vi "main.vi"(8 "Error in":errorcluster) -> (0 "error out":errorcluster)   [LabVIEW 2018, in "Controller.lvlib"]
doc: "The main VI of the module."
uses:
  Controller.lvlib
  vi/Module Queue Actions.ctl
  ctl/Module State--enum.ctl
  Common/Common.lvlib
  Common/ctl/Stop all modules states--enum.ctl
  Error Handler/Error Handler.lvlib
  Error Handler/ctl/Module State--enum.ctl
  Error Handler/ctl/Error source--enum.ctl
  Common/ctl/Error to pass.ctl
  Display Console/Simulated/Display Console.lvlib
  Sensor Interface/Simulated/Sensor Interface.lvlib
  User Console/Simulated/User Console.lvlib
  User Console/Simulated/ctl/Module State--enum.ctl
  vi/Module Data.ctl
  ctl/Module Data--cluster.ctl
  User Console/Simulated/ctl/control enable states--cluster.ctl
  Sensor Interface/Simulated/ctl/Module State--enum.ctl
  Display Console/Simulated/ctl/Module State--enum.ctl
  vi/state--global.vi
  ctl/Config db action--enum.ctl
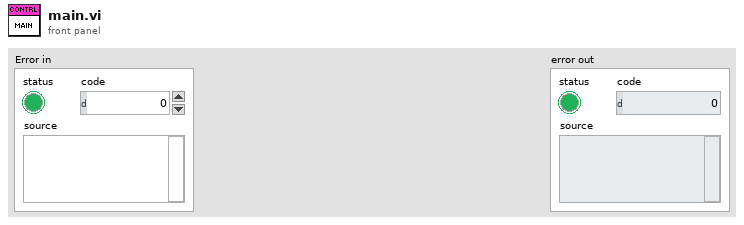
[diagram p1: front panel]
types:
  T1 = typedef "Controller.lvlib/Module Data--cluster.ctl" = cluster{"Atm messages":T2[], "No. incorrect login attempts":i32, "Balance":dbl}
  T2 = typedef "Controller.lvlib/Module Data.ctl" = cluster{"message name":string, "message text":string}
  T3 = typedef "Controller.lvlib/Module Queue Actions.ctl" = enum16{"Create", "Get", "Destroy"}
  T4 = typedef "Common.lvlib/Stop all modules states--enum.ctl" = enum16{"Create", "Get", "Send 'Stop all' Message", "Destroy"}
  T5 = typedef "Controller.lvlib/Module State--enum.ctl" = enum16{"Init", "Error", "Close", "User Console: Card Reader Pressed", "Sensor Interface: Deposit Received pressed", "Sensor Interface: Funds Dispensed Pressed", "Idle", "Login State", "Balance Enquiry", "Deposit State", "Withdrawal State", "Fast Cash State", "Configuration Database", "Inactivity Timeout", "Terminate State", "Wait for account number", "Verify account number", "Wait for new transaction button"}
  T6 = typedef "Common.lvlib/Error source--enum.ctl" = enum16{"Display Console", "User Console", "Sensor Interface IO", "Process Step", "Other"}
  T7 = typedef "Common.lvlib/Error to pass.ctl" = cluster{"Error source":T6, "Error":errorcluster}
  T8 = typedef "Error Handler.lvlib/Module State--enum.ctl" = enum16{"Init", "Error", "Idle", "Close", "Handle External Error", "Log to file"}
  T9 = typedef "User Console.lvlib/Module State--enum.ctl" = enum16{"Init", "Error", "Idle", "Close", "Transaction Button Pressed: Which?", "Balance Inquiry Pressed", "Desposit Pressed", "Withdrawal Pressed", "Fast Cash Pressed", "New Transaction Pressed", "Terminate Session Pressed", "Card Reader Pressed", "Keypad Button Pressed", "Update Keypad Screen", "Enable/disable controls", "Card reader: On?"}
  T10 = typedef "Display Console.lvlib/Module State--enum.ctl" = enum16{"Init", "Error", "Idle", "Close", "Card Read LED", "Update Message Screen", "Update Current Transaction", "Enable/disable controls"}
  T11 = typedef "Sensor Interface.lvlib/Module State--enum.ctl" = enum16{"Init", "Error", "Idle", "Close", "Enable/disable controls"}
  T12 = typedef "Controller.lvlib/Config db action--enum.ctl" = enum16{"Read", "Search", "Write"}
  T13 = typedef "User Console.lvlib/control enable states--cluster.ctl" = cluster{"Transactions":enum8{"Enabled", "Disabled", "Disabled and Grayed Out"}, "Card reader":enum8{"Enabled", "Disabled", "Disabled and Grayed Out"}, "Keypad":enum8{"Enabled", "Disabled", "Disabled and Grayed Out"}}
  T14 = typedef "Module Data.ctl" = cluster{"message name":string, "message text":string}
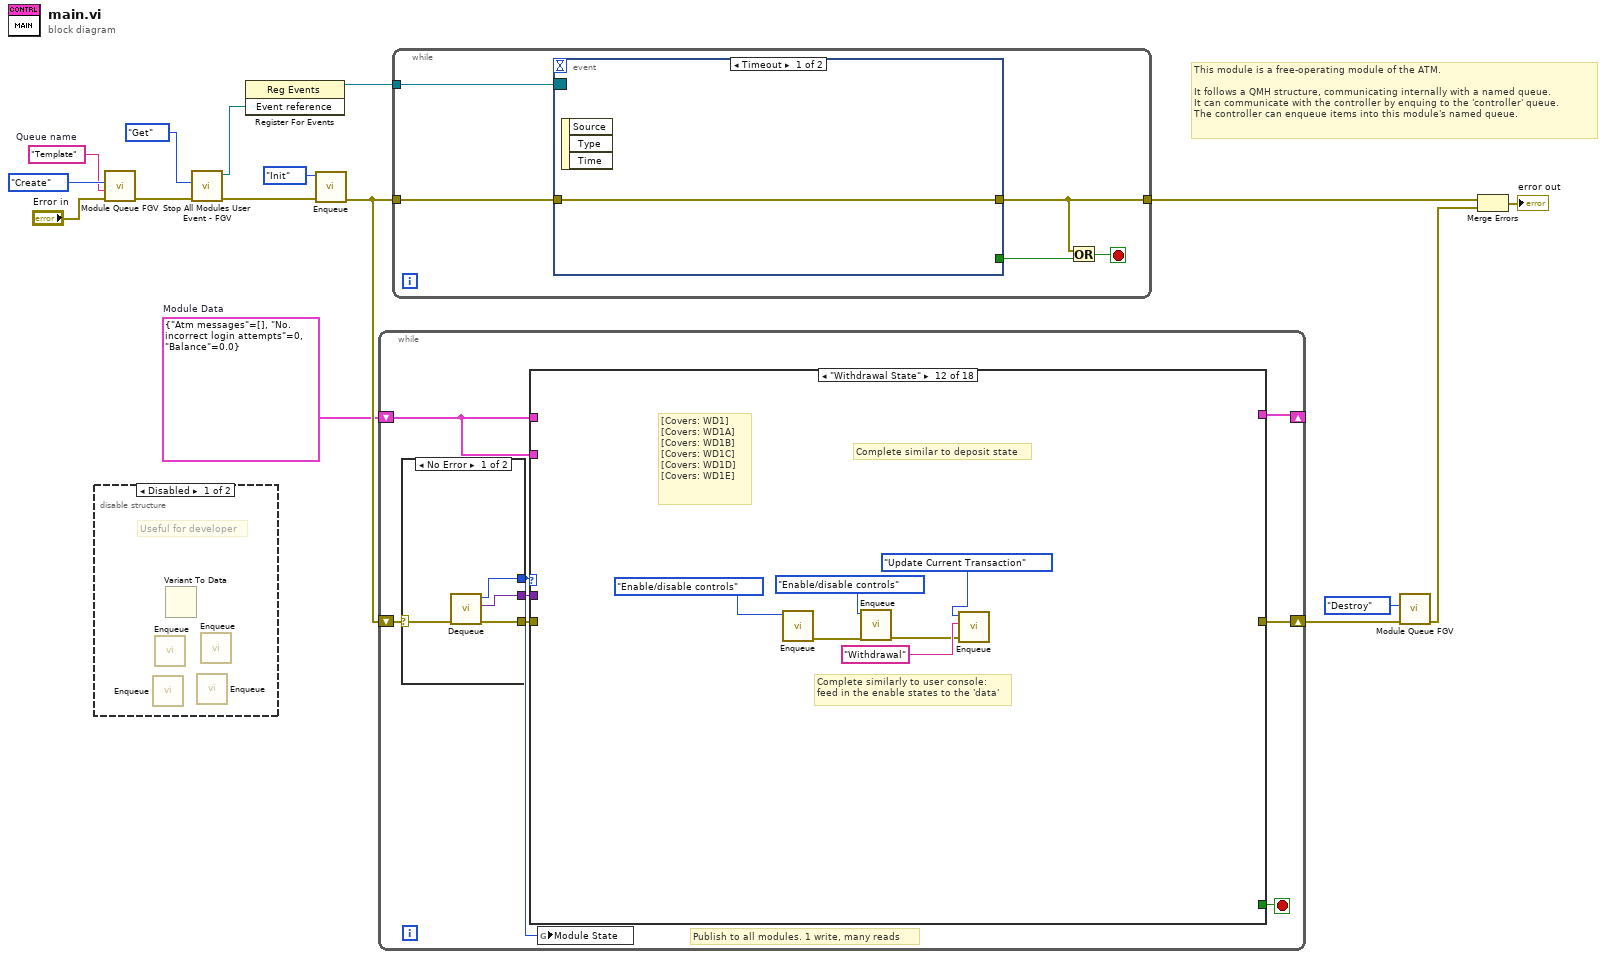
[diagram p0: block diagram]
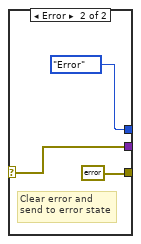
[diagram p3: hidden frame]
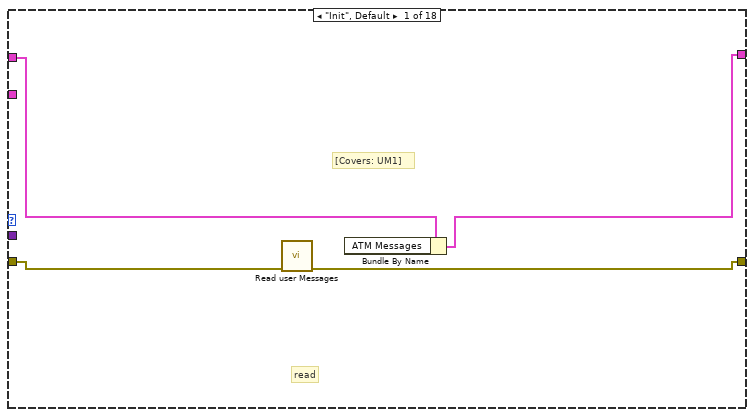
[diagram p4: hidden frame]
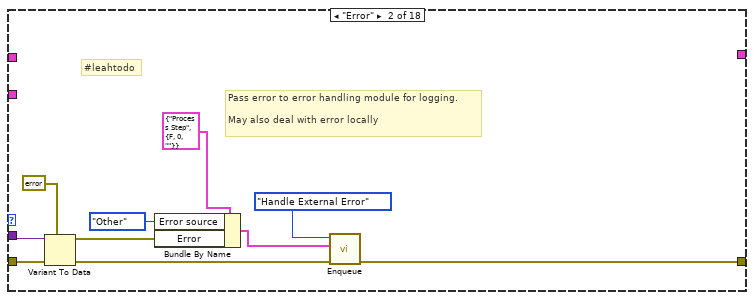
[diagram p5: hidden frame]
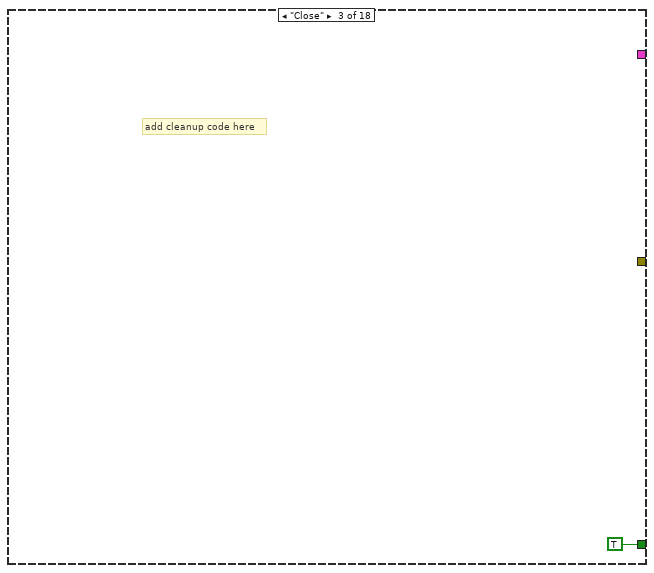
[diagram p6: hidden frame]
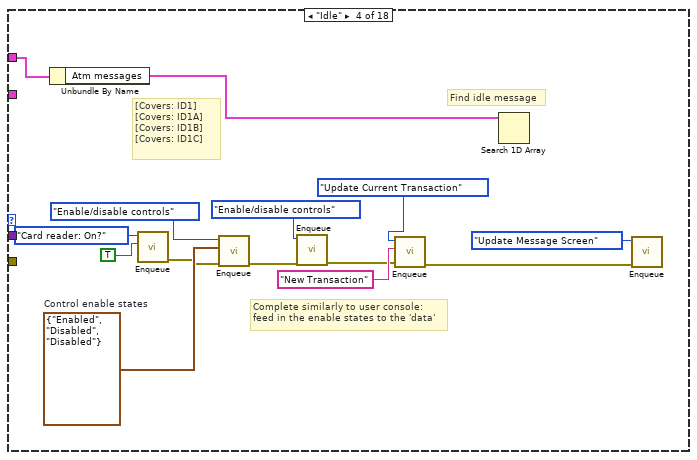
[diagram p7: hidden frame]
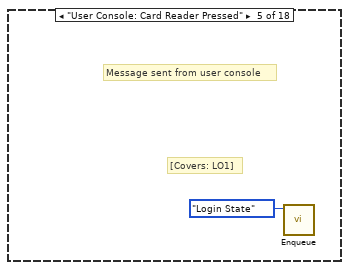
[diagram p8: hidden frame]
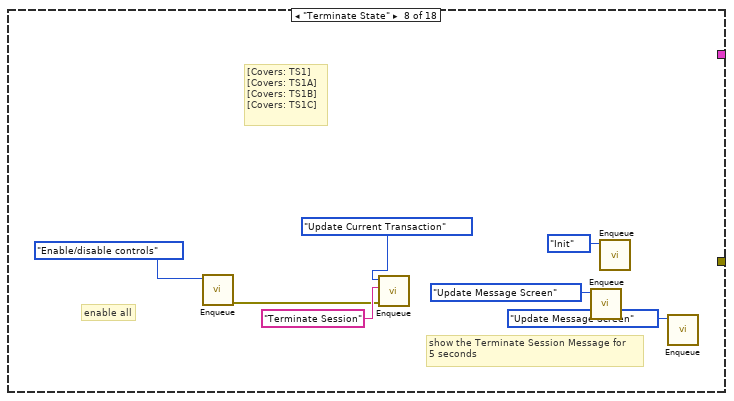
[diagram p11: hidden frame]
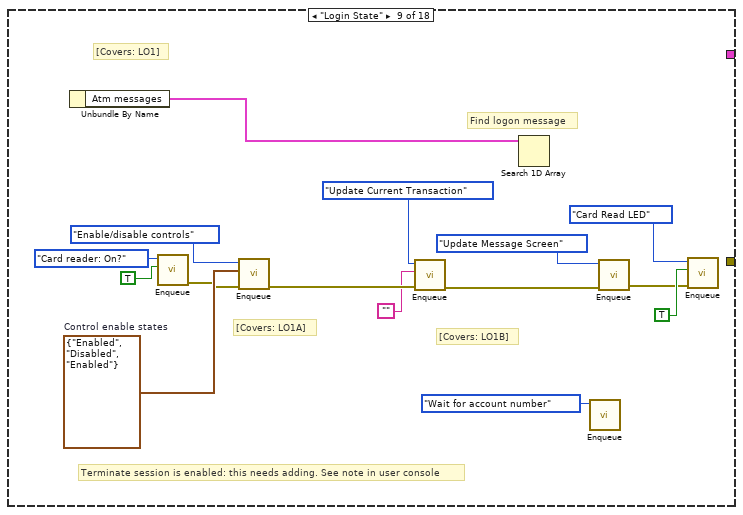
[diagram p12: hidden frame]
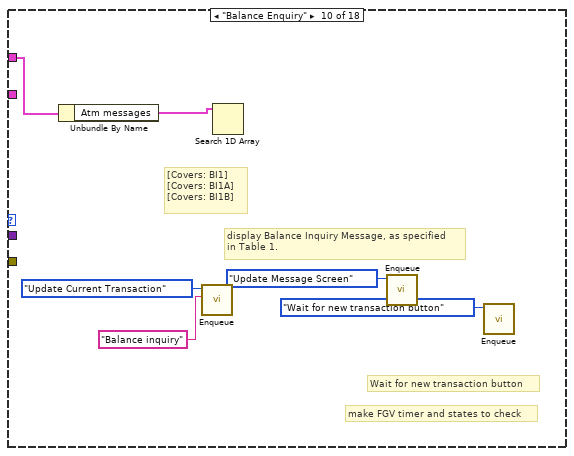
[diagram p13: hidden frame]
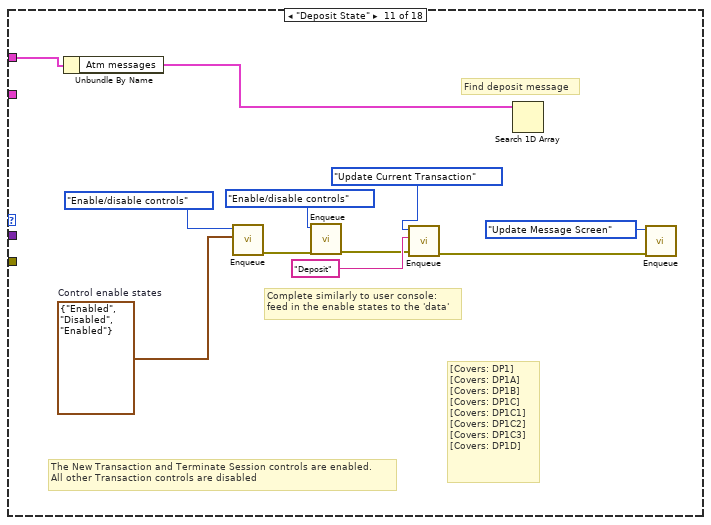
[diagram p14: hidden frame]
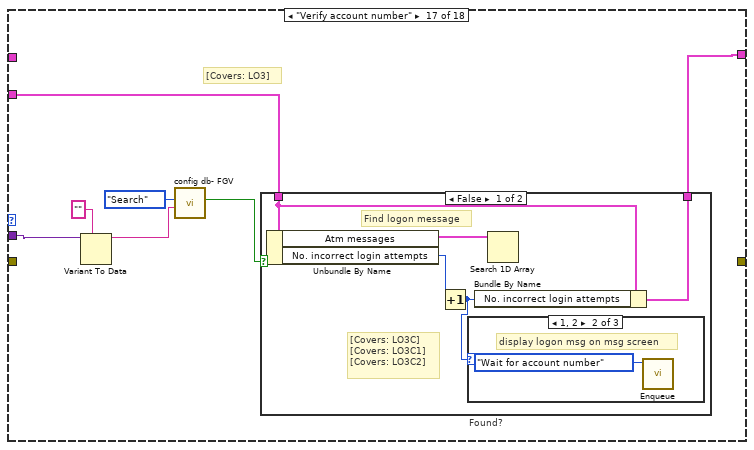
[diagram p19: hidden frame]
diagram:
  w1 = T1 {"Atm messages"=[], "No. incorrect login attempts"=0, "Balance"=0.0}  # Module Data
  w15 = "Template"  # Queue name
  # "This module is a free-operating module of the ATM.\n\nIt follows a QMH structure, communicating internally with a named queue.\nIt can communicate with the controller by enquing to the 'controller' queue.\nThe controller can enqueue items into this module's named queue."
  n1 = disable-structure shown="Disabled" {
    frame Disabled {
      # "Useful for developer"
      n2 = call "Enqueue.vi"() -> ()  [unwired: 11 in, 1 out]
      n3 = call "Enqueue.vi"() -> ()  [unwired: 11 in, 1 out]
      n4 = Variant To Data() -> ()  [unwired: 3 in, 2 out]
      n5 = call "Enqueue.vi"() -> ()  [unwired: 11 in, 1 out]
      n6 = call "Enqueue.vi"() -> ()  [unwired: 11 in, 1 out]
    }
    frame Enabled {
    }
  }
  n7 = call "Module Queue FGV.vi"("Error in"="Error in", "Queue name"=w15, "Module Queue Actions"=Module_Queue_Actions."Create") -> ("error out"=w10:errorcluster)  [unwired: 7 in, 1 out]
  n8 = call "Stop All Modules User Event - FGV.vi"("error in"=w10, "Action"=Stop_all_modules_states--enum."Get") -> ("error out"=w9:errorcluster, "Event reference"=w12:refnum<user-event>)  [unwired: 8 in]
  n9 = register-events(w12) -> (reference out=w11:refnum<event-registration>)  [unwired: 2 in, 1 out]
  n10 = call "Enqueue.vi"("error in (no error)"=w9, "State"=Module_State--enum."Init") -> ("error out"=w8:errorcluster)  [unwired: 9 in]
  n11 = while {
    shift-right: [w22] -> w6
    shift-left: w8 -> [w21]
    shift-right: [w19] -> _
    shift-left: w1 -> [w17]
    stop <- w20 stop-if-true
    # "Publish to all modules. 1 write, many reads"
    n12 = case shown="No Error" w21 {
      selector: w21 -> [w25 w30]
      tunnel: [w28 Module_State--enum."Error" ("State")] -> w18
      tunnel: [w27 w30] -> w24
      tunnel: [w26 errorcluster {"status"=FALSE, "code"=0, "source"=""} ("error out")] -> w23
      frame No Error {
        n13 = call "Dequeue.vi"("error in (no error)"=w25) -> ("error out"=w26:errorcluster, "Data"=w27:variant, "State"=w28:T5)  [unwired: 8 in]
      }
      frame Error {
        # "Clear error and\nsend to error state"
      }
    }
    n14 = case shown="\"Withdrawal State\"" w18 {
      tunnel: w24 -> [_ w42 _ _ _ _ _ _ _ _ _ _ _ _ _ _ w113 _]
      tunnel: w23 -> [w33 w43 _ _ _ _ _ _ _ _ _ _ _ _ _ _ _ _]
      tunnel: [w32 w44 _ _ _ _ _ _ _ _ _ _ _ _ _ _ _ _] -> w22
      tunnel: [_ _ TRUE _ _ _ _ _ _ _ _ _ _ _ _ _ _ _] -> w20
      tunnel: [w35 _ _ _ _ _ _ _ _ _ _ _ _ _ _ _ w107 _] -> w19
      tunnel: w17 -> [w34 _ _ w55 _ _ _ _ _ w86 w90 _ _ _ _ _ _ _]
      tunnel: w17 -> [_ _ _ _ _ _ _ _ _ _ _ _ _ _ _ _ w108 _]
      frame "Init", Default {
        # "[Covers: UM1]"
        # "read"
        n15 = call "Read user Messages.vi"("error in (no error)"=w33) -> ("error out"=w32:errorcluster)  [unwired: 9 in, 1 out]
        n16 = Bundle By Name(cluster=w34) -> (w35:T1)  [unwired: 1 in]
      }
      frame "Error" {
        # "#leahtodo"
        # "Pass error to error handling module for logging.\n\nMay also deal with error locally"
        n17 = Variant To Data(error in=w43, type=errorcluster {"status"=FALSE, "code"=0, "source"=""} ("error constant"), Variant=w42) -> (data=w38:errorcluster, error out=w40:errorcluster)
        n18 = Bundle By Name(cluster=T7 {"Error source"=enum."Process Step", "Error"={"status"=FALSE, "code"=0, "source"=""}} ("Error to pass"), "Error source"=Error_source--enum."Other", "Error"=w38) -> (w37:T7)
        n19 = call "Enqueue.vi"("error in (no error)"=w40, "Data"=w37, "State"=Module_State--enum."Handle External Error") -> ("error out"=w44:errorcluster)  [unwired: 8 in]
      }
      frame "Close" {
        # "add cleanup code here"
      }
      frame "Idle" {
        w59 = T13 {"Transactions"=enum."Enabled", "Card reader"=enum."Disabled", "Keypad"=enum."Disabled"}  # Control enable states
        # "Find idle message"
        # "Complete similarly to user console:\nfeed in the enable states to the 'data'"
        # "[Covers: ID1] \n[Covers: ID1A]   \n[Covers: ID1B] \n[Covers: ID1C]"
        n20 = Unbundle By Name(w55) -> ("Atm messages"=w53:T2[])
        n21 = call "Enqueue.vi"("Data"=TRUE, "State"=Module_State--enum."Card reader: On?") -> ("error out"=w50:errorcluster)  [unwired: 9 in]
        n22 = call "Enqueue.vi"("error in (no error)"=w50, "Data"=w59, "State"=Module_State--enum."Enable/disable controls") -> ("error out"=w49:errorcluster)  [unwired: 8 in]
        n23 = call "Enqueue.vi"("error in (no error)"=w49, "State"=Module_State--enum."Enable/disable controls") -> ("error out"=w48:errorcluster)  [unwired: 9 in]
        n24 = call "Enqueue.vi"("error in (no error)"=w48, "Data"="New Transaction", "State"=Module_State--enum."Update Current Transaction") -> ("error out"=w47:errorcluster)  [unwired: 8 in]
        n25 = Search 1D Array(1D array=w53) -> ()  [unwired: 2 in, 1 out]
        n26 = call "Enqueue.vi"("error in (no error)"=w47, "State"=Module_State--enum."Update Message Screen") -> ()  [unwired: 9 in, 1 out]
      }
      frame "User Console: Card Reader Pressed" {
        # "[Covers: LO1]"
        # "Message sent from user console"
        n27 = call "Enqueue.vi"("State"=Module_State--enum."Login State") -> ()  [unwired: 10 in, 1 out]
      }
      frame "Sensor Interface: Deposit Received pressed" {
      }
      frame "Sensor Interface: Funds Dispensed Pressed" {
      }
      frame "Terminate State" {
        # "enable all"
        # "show the Terminate Session Message for\n5 seconds"
        # "[Covers: TS1] \n[Covers: TS1A] \n[Covers: TS1B] \n[Covers: TS1C]"
        n28 = call "Enqueue.vi"("State"=Module_State--enum."Enable/disable controls") -> ("error out"=w65:errorcluster)  [unwired: 10 in]
        n29 = call "Enqueue.vi"("error in (no error)"=w65, "Data"="Terminate Session", "State"=Module_State--enum."Update Current Transaction") -> ()  [unwired: 8 in, 1 out]
        n30 = call "Enqueue.vi"("State"=Module_State--enum."Update Message Screen") -> ()  [unwired: 10 in, 1 out]
        n31 = call "Enqueue.vi"("State"=Module_State--enum."Init") -> ()  [unwired: 10 in, 1 out]
        n32 = call "Enqueue.vi"("State"=Module_State--enum."Update Message Screen") -> ()  [unwired: 10 in, 1 out]
      }
      frame "Login State" {
        w82 = T13 {"Transactions"=enum."Enabled", "Card reader"=enum."Disabled", "Keypad"=enum."Enabled"}  # Control enable states
        # "[Covers: LO1A]"
        # "[Covers: LO1B]"
        # "Terminate session is enabled: this needs adding. See note in user console"
        # "Find logon message"
        # "[Covers: LO1]"
        n33 = Unbundle By Name() -> ("Atm messages"=w79:T14[])  [unwired: 1 in]
        n34 = call "Enqueue.vi"("Data"=TRUE, "State"=Module_State--enum."Card reader: On?") -> ("error out"=w76:errorcluster)  [unwired: 9 in]
        n35 = call "Enqueue.vi"("error in (no error)"=w76, "Data"=w82, "State"=Module_State--enum."Enable/disable controls") -> ("error out"=w75:errorcluster)  [unwired: 8 in]
        n36 = call "Enqueue.vi"("error in (no error)"=w75, "Data"="", "State"=Module_State--enum."Update Current Transaction") -> ("error out"=w74:errorcluster)  [unwired: 8 in]
        n37 = Search 1D Array(1D array=w79) -> ()  [unwired: 2 in, 1 out]
        n38 = call "Enqueue.vi"("State"=Module_State--enum."Wait for account number") -> ()  [unwired: 10 in, 1 out]
        n39 = call "Enqueue.vi"("error in (no error)"=w74, "State"=Module_State--enum."Update Message Screen") -> ("error out"=w70:errorcluster)  [unwired: 9 in]
        n40 = call "Enqueue.vi"("error in (no error)"=w70, "Data"=TRUE, "State"=Module_State--enum."Card Read LED") -> ()  [unwired: 8 in, 1 out]
      }
      frame "Balance Enquiry" {
        # "Wait for new transaction button"
        # "display Balance Inquiry Message, as specified\nin Table 1."
        # "make FGV timer and states to check"
        # "[Covers: BI1] \n[Covers: BI1A] \n[Covers: BI1B]"
        n41 = Unbundle By Name(w86) -> ("Atm messages"=w85:T2[])
        n42 = call "Enqueue.vi"("Data"="Balance inquiry", "State"=Module_State--enum."Update Current Transaction") -> ()  [unwired: 9 in, 1 out]
        n43 = Search 1D Array(1D array=w85) -> ()  [unwired: 2 in, 1 out]
        n44 = call "Enqueue.vi"("State"=Module_State--enum."Update Message Screen") -> ()  [unwired: 10 in, 1 out]
        n45 = call "Enqueue.vi"("State"=Module_State--enum."Wait for new transaction button") -> ()  [unwired: 10 in, 1 out]
      }
      frame "Deposit State" {
        w99 = T13 {"Transactions"=enum."Enabled", "Card reader"=enum."Disabled", "Keypad"=enum."Enabled"}  # Control enable states
        # "[Covers: DP1] \n[Covers: DP1A] \n[Covers: DP1B] \n[Covers: DP1C] \n[Covers: DP1C1] \n[Covers: DP1C2] \n[Covers: DP1C3] \n[Covers: DP1D]"
        # "The New Transaction and Terminate Session controls are enabled.\nAll other Transaction controls are disabled"
        # "Find deposit message"
        # "Complete similarly to user console:\nfeed in the enable states to the 'data'"
        n46 = Unbundle By Name(w90) -> ("Atm messages"=w94:T2[])
        n47 = call "Enqueue.vi"("Data"=w99, "State"=Module_State--enum."Enable/disable controls") -> ("error out"=w93:errorcluster)  [unwired: 9 in]
        n48 = call "Enqueue.vi"("error in (no error)"=w93, "State"=Module_State--enum."Enable/disable controls") -> ("error out"=w92:errorcluster)  [unwired: 9 in]
        n49 = call "Enqueue.vi"("error in (no error)"=w92, "Data"="Deposit", "State"=Module_State--enum."Update Current Transaction") -> ("error out"=w91:errorcluster)  [unwired: 8 in]
        n50 = Search 1D Array(1D array=w94) -> ()  [unwired: 2 in, 1 out]
        n51 = call "Enqueue.vi"("error in (no error)"=w91, "State"=Module_State--enum."Update Message Screen") -> ()  [unwired: 9 in, 1 out]
      }
      frame "Withdrawal State" {
        # "Complete similar to deposit state"
        # "[Covers: WD1] \n[Covers: WD1A]  \n[Covers: WD1B] \n[Covers: WD1C] \n[Covers: WD1D]\n[Covers: WD1E]"
        # "Complete similarly to user console:\nfeed in the enable states to the 'data'"
        n52 = call "Enqueue.vi"("State"=Module_State--enum."Enable/disable controls") -> ("error out"=w102:errorcluster)  [unwired: 10 in]
        n53 = call "Enqueue.vi"("error in (no error)"=w102, "State"=Module_State--enum."Enable/disable controls") -> ("error out"=w101:errorcluster)  [unwired: 9 in]
        n54 = call "Enqueue.vi"("error in (no error)"=w101, "Data"="Withdrawal", "State"=Module_State--enum."Update Current Transaction") -> ()  [unwired: 8 in, 1 out]
      }
      frame "Fast Cash State" {
      }
      frame "Configuration Database" {
      }
      frame "Inactivity Timeout" {
      }
      frame "Wait for account number" {
        # "message comes from user console"
      }
      frame "Verify account number" {
        # "[Covers: LO3]"
        n55 = Variant To Data(type="", Variant=w113) -> (data=w110:string)  [unwired: 1 in, 1 out]
        n56 = call "config db- FGV.vi"("Search string"=w110, "Action"=Config_db_action--enum."Search") -> ("Found?"=w109:bool)  [unwired: 8 in, 1 out]
        n57 = case "Found?" shown="False" w109 {
          tunnel: w108 -> [w117 w121]
          tunnel: [w116 w121] -> w107
          frame False {
            # "[Covers: LO3C] \n[Covers: LO3C1] \n[Covers: LO3C2]"
            # "Find logon message"
            n58 = Unbundle By Name(w117) -> ("Atm messages"=w118:T2[], "No. incorrect login attempts"=w115:i32)
            n59 = Increment(x=w115) -> (x+1=w114:i32)
            n60 = case shown="1, 2" w114 {
              frame Default {
              }
              frame 1, 2 {
                # "display logon msg on msg screen"
                n61 = call "Enqueue.vi"("State"=Module_State--enum."Wait for account number") -> ()  [unwired: 10 in, 1 out]
              }
              frame 3 {
                n62 = call "Enqueue.vi"("State"=Module_State--enum."Terminate State") -> ()  [unwired: 10 in, 1 out]
              }
            }
            n63 = Bundle By Name(cluster=w117, "No. incorrect login attempts"=w114) -> (w116:T1)
            n64 = Search 1D Array(1D array=w118) -> ()  [unwired: 2 in, 1 out]
          }
          frame True {
            # "[Covers: LO3A]"
            n65 = call "Enqueue.vi"("State"=Module_State--enum."Idle") -> ()  [unwired: 10 in, 1 out]
          }
        }
      }
      frame "Wait for new transaction button" {
        # "[Covers: BI1B]"
        # "5 seconds goal"
        # "make FGV timer and keep looping check state"
        n66 = And() -> (x .and. y?=w123:bool)  [unwired: 2 in]
        n67 = case "time elapsed?" shown="True" w123 {
          frame False {
          }
          frame True {
            n68 = call "Enqueue.vi"("State"=Module_State--enum."Idle") -> ()  [unwired: 10 in, 1 out]
          }
        }
      }
    }
    n69 = global write "state--global.vi" "Module State"(w18) -> ()
  }
  n70 = while {
    tunnel: w8 -> [w129]
    tunnel: [w126] -> w4
    tunnel: w11 -> [w128]
    stop <- w127 stop-if-true
    n71 = event shown="[0] Timeout" {
      selector: w128 -> [_ _]
      dyn-events: _ -> [_ _]
      timeout: _ -> [_ _]
      tunnel: w129 -> [w130 w134]
      tunnel: [w130 w133] -> w126
      tunnel: [_ TRUE] -> w125
      event Timeout {
        n72 = event-data() -> ()  [unwired: 1 in, 3 out]
      }
      event User Event {
        # "Stop message has been received - shut down"
        n73 = event-data() -> ()  [unwired: 1 in, 1 out]
        n74 = call "Enqueue.vi"("error in (no error)"=w134, "State"=Module_State--enum."Close") -> ("error out"=w133:errorcluster)  [unwired: 9 in]
      }
    }
    n75 = Or(x=w126, y=w125) -> (x .or. y?=w127:bool)
  }
  n76 = call "Module Queue FGV.vi"("Error in"=w6, "Module Queue Actions"=Module_Queue_Actions."Destroy") -> ("error out"=w5:errorcluster)  [unwired: 8 in, 1 out]
  n77 = Merge Errors(w4, w5) -> (→"error out":errorcluster)
